vi "Get_Refresh_Token.vi"(8 "error in (no error)":errorcluster, 11 "OneNote in":refnum<class "OneNote.lvclass">) -> (0 "error out":errorcluster, 3 "OneNote out":refnum<class "OneNote.lvclass">)   [LabVIEW 2016, in "OneNote.lvclass"]
uses:
  OneNote.lvclass
  OAuth/OAuth.lvclass
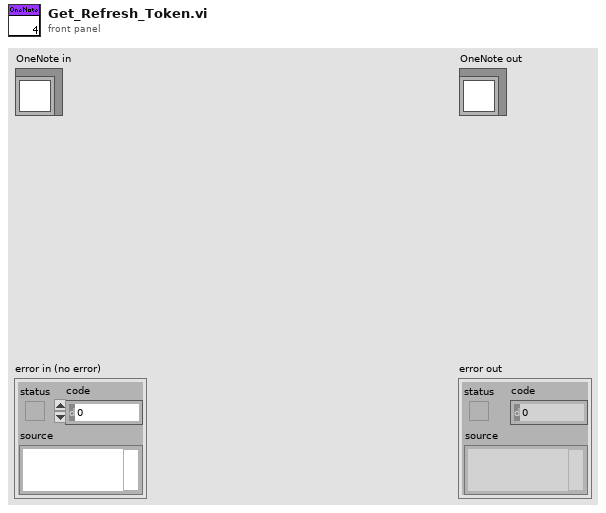
[diagram p1: front panel]
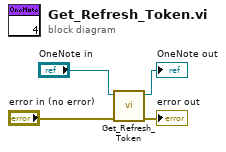
[diagram p0: block diagram]
diagram:
  n1 = call-parent "Get_Refresh_Token.vi"("error in (no error)"="error in (no error)", "OAuth in"="OneNote in") -> ("error out"=→"error out":errorcluster, "OAuth out"=→"OneNote out":refnum<class "OneNote.lvclass">)  [unwired: 8 in]
